vi "dfd_NStage MRate Filter Design with FIR.vi"(5 "fs [Hz]":dbl=1000.0, 6 "filtering mode":T8=2 items=["No Rate Change", "Interpolation", "Decimation"], 8 "error in":errorcluster, 9 "ripple specs":T2={"passband"=0.05437453093312722, "stopband"=0.001, "dB/linear? (T: dB)"=FALSE}, 10 "freq spec":T1={"fpass"=55.0, "fstop"=70.0}, 11 "current factor":i32=2) -> (0 "error out":errorcluster, 3 "multirate filter out":T3={"mMRate_Structure"=enum."FIR", "mMRate_Mode"=2, "mMRate_Factor"=2, "mMRate_FIRParams"={"mMRate_FIR_H"=[0.06643225836299978, 0.25769958342885607, 0.38221664117622445, 0.25769958342885607, 0.06643225836299978], "mMRate_FIR_IsNyquist?"=FALSE, "mMRate_FIR_IsSymmetric?"=FALSE}, "mMRate_CICParams"={"mMRate_CIC_#Stage"=2, "mMRate_CIC_Lag"=1, "mMRate_CIC_Type"=enum."Lowpass"}, "mMRate_Order"=4, "mMRate_Version"="1.0", "mMRate_Comments"="1.0", "mMRate_RationalFactor"={"mMRate_L"=-1, "mMRate_M"=-1}, "mMRate_Fs"=1.0, "mMRate_Quantized?"=FALSE, "mMRate_QFilterGain"=1.0, "mMRate_CoefWl"=16, "mMRate_Scaling"={"mMRate_ScaleByPowerOf2?"=FALSE, "mMRate_ScaleType"=enum."Time Domain 1-Norm"}, "mMRate_InputWl"=0, "mMRate_OutputWl"=0, "mMRate_OutputMode"=enum."Nearest", "mMRate_MultMode"=enum."Full", "mMRate_BitPruning"=FALSE, "mMRate_GainWl"=16, "mMRate_OutputFwl"=0, "mMRate_SumIwl"=0, "mMRate_InputIwl "=16, "mMRate_SumWl"=32, "mMRate_CoefIwl"=0} {"mMRate_SumWl" min=1 max=32 step=1; "mMRate_InputIwl" min=1 max=32 step=1; "mMRate_GainWl" min=1 max=32 step=1; "mMRate_OutputWl" min=1 max=32 step=1; "mMRate_InputWl" min=1 max=32 step=1; "mMRate_CoefWl" min=1 max=32 step=1; "mMRate_Mode" items=["Default"=-1, "No Rate Change"=0, "Interpolation"=1, "Decimation"=2, "Interpolated"=3, "Rational"=4]})   [LabVIEW 2017, in "NI_DigFilterLicensed.lvlib"]
uses:
  <vilib>/addons/Digital Filter Design/NI_DigFilterLicensed.lvlib
  <vilib>/addons/Digital Filter Design/_Objects.llb/DFD Multirate Filtering Mode.ctl
  <vilib>/addons/Digital Filter Design/_Objects.llb/DFD Multirate Filter Obj.ctl
  <vilib>/addons/Digital Filter Design/_Objects.llb/DFD Multirate Mode.ctl
  <vilib>/addons/Digital Filter Design/_Objects.llb/DFD Coef Norm Type.ctl
  <vilib>/addons/Digital Filter Design/_Objects.llb/DFD Round-off Mode.ctl
  <vilib>/addons/Digital Filter Design/_Objects.llb/DFD FXP MRate Multiply Mode.ctl
  <vilib>/addons/Digital Filter Design/_Objects.llb/DFD Filter Ripple Specification (Design).ctl
  <vilib>/addons/Digital Filter Design/_Objects.llb/DFD Multirate Filter Specification (Design).ctl
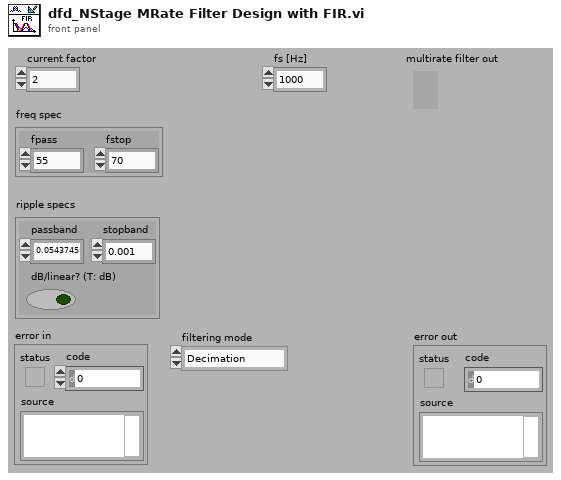
[diagram p1: front panel]
types:
  T1 = typedef "NI_DigFilterLicensed.lvlib/DFD Multirate Filter Specification (Design).ctl" = cluster{"fpass":dbl, "fstop":dbl}
  T2 = typedef "NI_DigFilterLicensed.lvlib/DFD Filter Ripple Specification (Design).ctl" = cluster{"passband":dbl, "stopband":dbl, "dB/linear? (T: dB)":bool}
  T3 = typedef "NI_DigFilterLicensed.lvlib/DFD Multirate Filter Obj.ctl" = cluster{"mMRate_Structure":enum16{"CIC", "FIR", "IIR", "Lattice"}, "mMRate_Mode":T4, "mMRate_Factor":i32, "mMRate_FIRParams":cluster{"mMRate_FIR_H":dbl[], "mMRate_FIR_IsNyquist?":bool, "mMRate_FIR_IsSymmetric?":bool}, "mMRate_CICParams":cluster{"mMRate_CIC_#Stage":i32, "mMRate_CIC_Lag":i32, "mMRate_CIC_Type":enum16{"Lowpass", "Highpass"}}, "mMRate_Order":i32, "mMRate_Version":string, "mMRate_Comments":string, "mMRate_RationalFactor":cluster{"mMRate_L":i32, "mMRate_M":i32}, "mMRate_Fs":dbl, "mMRate_Quantized?":bool, "mMRate_QFilterGain":dbl, "mMRate_CoefWl":i16, "mMRate_Scaling":cluster{"mMRate_ScaleByPowerOf2?":bool, "mMRate_ScaleType":T5}, "mMRate_InputWl":i16, "mMRate_OutputWl":i16, "mMRate_OutputMode":T6, "mMRate_MultMode":T7, "mMRate_BitPruning":bool, "mMRate_GainWl":i16, "mMRate_OutputFwl":i16, "mMRate_SumIwl":i16, "mMRate_InputIwl ":i16, "mMRate_SumWl":i16, "mMRate_CoefIwl":i16}
  T4 = typedef "NI_DigFilterLicensed.lvlib/DFD Multirate Mode.ctl" = i16
  T5 = typedef "NI_DigFilterLicensed.lvlib/DFD Coef Norm Type.ctl" = enum16{"No Norm", "Time Domain 1-Norm", "Time Domain 2-Norm", "Time Domain Inf-Norm"}
  T6 = typedef "NI_DigFilterLicensed.lvlib/DFD Round-off Mode.ctl" = enum16{"Nearest", "Truncation"}
  T7 = typedef "NI_DigFilterLicensed.lvlib/DFD FXP MRate Multiply Mode.ctl" = enum16{"Truncated", "Full"}
  T8 = typedef "NI_DigFilterLicensed.lvlib/DFD Multirate Filtering Mode.ctl" = u16
  T9 = enum16{"Lowpass", "Highpass", "Bandpass", "Bandstop"}
  T10 = enum16{"Butterworth", "Chebyshev", "Inverse Chebyshev", "Elliptic", "Kaiser Window", "Dolph-Chebyshev Window", "Equi-Ripple FIR"}
  T11 = typedef "NI_DigFilterLicensed.lvlib/DFD Filter Obj.ctl" = cluster{"mSRate_Fs":dbl, "mSRate_Version":string, "mSRate_Comments":string, "mSRate_OrgCoef":T12, "mSRate_CurCoef":T12, "mSRate_Quantized?":bool, "mSRate_QCoef":T12, "mSRate_QSettings":T14[], "mSRate_Order":i32, "mSRate_Scaling":cluster{"mSRate_ScaleByPowerOf2?":bool, "mSRate_ScaleType":T5}}
  T12 = typedef "NI_DigFilterLicensed.lvlib/DFD Filter Coef.ctl" = cluster{"type":T13, "gain":dbl, "coef a (k)":dbl[], "coef b (v)":dbl[]}
  T13 = typedef "NI_DigFilterLicensed.lvlib/DFD Filter Structure Type Selector.ctl" = enum16{"Undefined", "FIR Direct Form", "FIR Direct Form Transposed", "FIR Symmetric", "FIR Antisymmetric", "IIR Direct Form I", "IIR Direct Form I Transposed", "IIR Direct Form II", "IIR Direct Form II Transposed", "IIR Cascaded Second Order Sections Form I", "IIR Cascaded Second Order Sections Form I Transposed", "IIR Cascaded Second Order Sections Form II", "IIR Cascaded Second Order Sections Form II Transposed", "Lattice Allpass (basic sections)", "Lattice Allpass (one multiplier sections)", "Lattice Allpass (normalized sections)", "Lattice AR (basic sections)", "Lattice AR (one multiplier sections)", "Lattice AR (normalized sections)", "Lattice MA (minimum phase)", "Lattice MA (maximum phase)", "Lattice ARMA (basic sections)", "Lattice ARMA (one multiplier sections)", "Lattice ARMA (normalized sections)"}
  T14 = typedef "NI_DigFilterLicensed.lvlib/dfd_Internal Quantization Settings.ctl" = cluster{"source":T15, "wl":i16, "iwl":i16, "overflow mode":enum16{"Saturation", "Wrap"}, "rounding mode":enum16{"Nearest", "Truncation"}, "signed?":bool}
  T15 = typedef "NI_DigFilterLicensed.lvlib/dfd_Internal Quantization Srcs.ctl" = u16
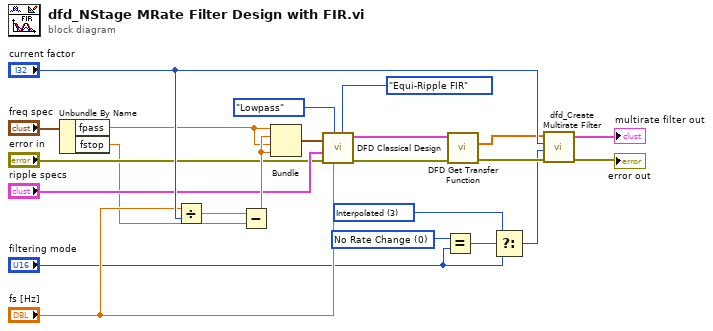
[diagram p0: block diagram]
diagram:
  w3 = T4 3 items=["Default"=-1, "No Rate Change"=0, "Interpolation"=1, "Decimation"=2, "Interpolated"=3, "Rational"=4] ("mode")
  w5 = T8 0 items=["No Rate Change", "Interpolation", "Decimation"] ("x")
  n1 = Unbundle By Name("freq spec") -> ("fpass"=w7:dbl, "fstop"=w6:dbl)
  n2 = Divide(x="fs [Hz]", y="current factor") -> (x/y=w16:dbl)
  n3 = Subtract(x=w16, y=w6) -> (x-y=w18:dbl)
  n4 = Bundle("fpass"=w7, w18, "fpass"=w7, w18) -> (w19:cluster{"fpass":dbl, dbl, "fpass":dbl, dbl})  [unwired: 1 out]
  n5 = call <vilib>:"DFD Classical Design.vi"("design method"=T10."Equi-Ripple FIR", "fs [Hz]"="fs [Hz]", "filter type"=T9."Lowpass", "error in (no error)"="error in", "ripple specs"="ripple specs", "freq specs [Hz]"=w19) -> ("error out"=w11:errorcluster, "filter out"=w22:T11)  [unwired: 4 out]
  n6 = Equal?(x=w5, y="filtering mode") -> (x = y?=w4:bool)
  n7 = call <vilib>:"DFD Get Transfer Function.vi"("error in (no error)"=w11, "filter in"=w22) -> ("error out"=w12:errorcluster, "numerator"=w13:dbl[])  [unwired: 8 out]
  n8 = Select(t=w3, s=w4, f="filtering mode") -> (s? t:f=w1:T8)
  n9 = call <vilib>:"dfd_Create Multirate Filter.vi"("error in (no error)"=w12, "mode"=w1, "factor"="current factor", "h (n)"=w13) -> ("error out"=→"error out":errorcluster, "multirate filter out"=→"multirate filter out":T3)  [unwired: 1 in, 5 out]
